vi "频率.vi"() -> ()   [LabVIEW 2010]
panel:
  in  "频率":dbl=400.0
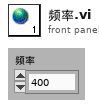
[diagram p1: front panel]
diagram:
